vi "Terminal-GearSystem-SelfCheck.vi"(8 "error in (no error)":errorcluster caption="错误输入（无错误）") -> (0 "error out":errorcluster caption="错误输出")   [LabVIEW 2014]
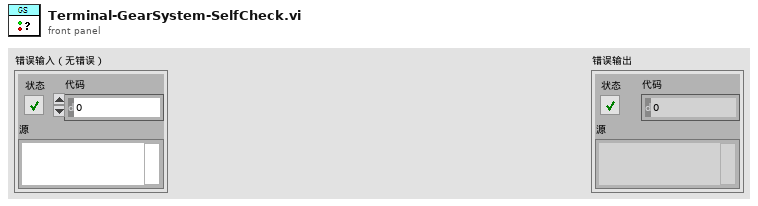
[diagram p1: front panel]
types:
  T1 = cluster{"油箱温度":u16, "供油油温":u16, "供油压力":u16, "油箱润滑油液位":bool, "1号油泵状态":bool, "2号油泵状态":bool, "回油泵状态":bool, "散热器风机状态":bool, "供油流量状态":bool, "过滤器压差":bool, "油箱系统综合状态":bool, "齿轮箱轴承温度1":u16, "齿轮箱轴承温度2":u16, "齿轮箱轴承温度3":u16, "齿轮箱轴承温度4":u16, "齿轮箱轴承温度5":u16, "齿轮箱轴承温度6":u16, "齿轮箱轴承温度7":u16, "齿轮箱轴承温度8":u16, "齿轮子系统状态字":cluster{"油箱加热器异常故障报警":bool, "油箱液位过高报警":bool, "油箱液位过低报警":bool, "供油过滤器压差过高报警":bool, "1号油泵故障报警":bool, "2号油泵故障报警":bool, "回油泵故障报警":bool, "散热器风机故障报警":bool, "供油压力异常报警":bool, "供油流量异常报警":bool, "供油油温异常报警":bool, "油站系统综合状态异常报警":bool, "轴承温度异常报警":bool}}
  T2 = cluster{"油箱加热器异常故障报警":bool, "油箱液位过高报警":bool, "油箱液位过低报警":bool, "供油过滤器压差过高报警":bool, "1号油泵故障报警":bool, "2号油泵故障报警":bool, "回油泵故障报警":bool, "散热器风机故障报警":bool, "供油压力异常报警":bool, "供油流量异常报警":bool, "供油油温异常报警":bool, "油站系统综合状态异常报警":bool, "轴承温度异常报警":bool}
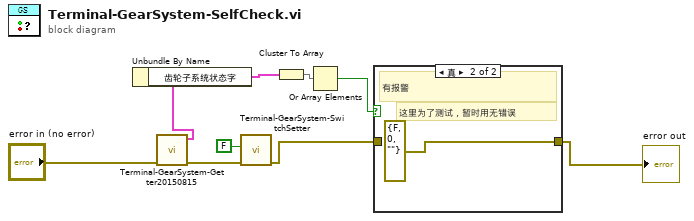
[diagram p0: block diagram]
diagram:
  n1 = call "Terminal-GearSystem-Getter20150815.vi"("error in (no error)"="error in (no error)") -> ("error out"=w8:errorcluster, "设备信息"=w6:T1)  [unwired: 8 in, 1 out]
  n2 = Unbundle By Name(w6) -> ("齿轮子系统状态字"=w5:T2)
  n3 = call "Terminal-GearSystem-SwitchSetter.vi"("error in (no error)"=w8, "启停"=FALSE) -> ("error out"=w4:errorcluster)  [unwired: 9 in]
  n4 = Cluster To Array(cluster=w5) -> (array=w2:bool[])
  n5 = Or Array Elements(Boolean array=w2) -> (logical OR=w1:bool)
  n6 = case shown="真" w1 {
    tunnel: [w10 errorcluster {"status"=FALSE, "code"=0, "source"=""} ("错误常量")] -> w3
    tunnel: w4 -> [w10 _]
    frame False {
      # "没有报警"
    }
    frame True {
      # "这里为了测试，暂时用无错误"
      # "有报警"
    }
  }
  "error out" <- w3
